vi "曲线生成.vi"(7 "YScale.Mapping Mode":u8, 9 "Y":dbl[](array[numeric]), 11 "X":dbl[](array[numeric])) -> (3 "曲线":cluster{dbl[], dbl[]}[](array[cluster]), 5 "突变电压":dbl)   [LabVIEW 2021]
uses:
  <vilib>/Analysis/NI_AALPro.lvlib
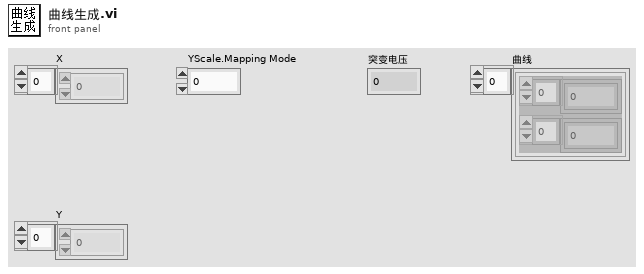
[diagram p1: front panel]
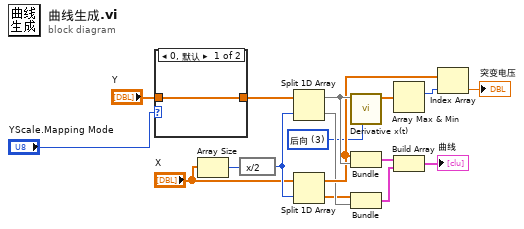
[diagram p0: block diagram]
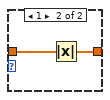
[diagram p2: hidden frame]
diagram:
  w1 = u16 3 items=["二阶中心", "四阶中心", "前向", "后向"] ("method")
  n1 = case shown="0, 默认" "YScale.Mapping Mode" {
    tunnel: "Y" -> [w18 w20]
    tunnel: [w18 w19] -> w14
    frame 0, Default {
    }
    frame 1 {
      n2 = Absolute Value(x=w20) -> (abs(x)=w19:dbl[])
    }
  }
  n3 = Array Size(array="X") -> (size(s)=w15:i32)
  n4 = expression code="x/2"(w15) -> (w16:i32)
  n5 = Split 1D Array(array=w14, index=w16) -> (first subarray=w17:dbl[], second subarray=w11:dbl[])
  n6 = Split 1D Array(array="X", index=w16) -> (first subarray=w12:dbl[], second subarray=w10:dbl[])
  n7 = call <vilib>:"Derivative x(t).vi"("method"=w1, "X"=w17) -> ("dX/dt"=w2:dbl[])  [unwired: 8 in, 1 out]
  n8 = Bundle(w12, w17) -> (w8:cluster{dbl[], dbl[]})  [unwired: 1 in]
  n9 = Bundle(w10, w11) -> (w9:cluster{dbl[], dbl[]})  [unwired: 1 in]
  n10 = Array Max & Min(array=w2) -> (max index (indices)=w13:i32)  [unwired: 3 out]
  n11 = Build Array(w8, w9) -> (→"曲线":cluster{dbl[], dbl[]}[])
  n12 = Index Array(array=w12, index=w13) -> (element=→"突变电压":dbl)
